vi "Voltages_2_U16.vi"(0 "Voltages":dbl[][](array[numeric])) -> (1 "Scale and Offset":T1(array[cluster]), 2 "U16 data":u16[][](array[numeric]))   [LabVIEW 2013]
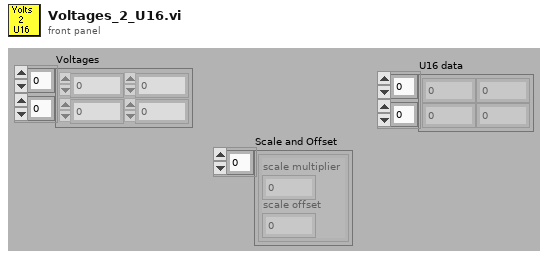
[diagram p1: front panel]
types:
  T1 = cluster{"scale multiplier":dbl, "scale offset":dbl}[]
  T2 = cluster{"scale multiplier":dbl, "scale offset":dbl}
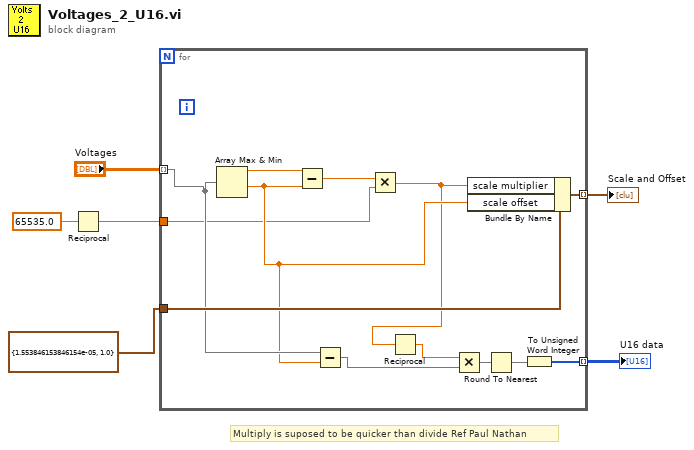
[diagram p0: block diagram]
diagram:
  # "Multiply is suposed to be quicker than divide Ref Paul Nathan"
  n1 = Reciprocal(x=65535.0 ("y")) -> (1/x=w1:dbl)
  n2 = for {
    tunnel: T2 {"scale multiplier"=1.553846153846154e-05, "scale offset"=1.0} -> [w19]
    tunnel: [w18] -> w5 mode=indexing
    tunnel: [w16] -> w4 mode=indexing
    tunnel: "Voltages" -> [w15] mode=indexing
    tunnel: w1 -> [w11]
    n3 = Array Max & Min(array=w15) -> (max value=w17:dbl, min value=w14:dbl)  [unwired: 2 out]
    n4 = Subtract(x=w17, y=w14) -> (x-y=w13:dbl)
    n5 = Subtract(x=w15, y=w14) -> (x-y=w8:dbl[])
    n6 = Multiply(x=w13, y=w11) -> (x*y=w10:dbl)
    n7 = Reciprocal(x=w10) -> (1/x=w9:dbl)
    n8 = Multiply(x=w9, y=w8) -> (x*y=w7:dbl[])
    n9 = Bundle By Name(cluster=w19, "scale multiplier"=w10, "scale offset"=w14) -> (w18:T2)
    n10 = Round To Nearest(number=w7) -> (nearest integer value=w12:dbl[])
    n11 = To Unsigned Word Integer(number=w12) -> (unsigned 16bit integer=w16:u16[])
  }
  "Scale and Offset" <- w5
  "U16 data" <- w4
